vi "MethodSCRIPTExample.vi"() -> ()   [LabVIEW 2025]
uses:
  PalmSens/PalmSens.lvclass
  PalmSens/MeasurementResults.ctl
  PalmSens/LiveCurveResult.ctl
  C:/Users/stef/code/palmsenssdk/labview/PalmSens/Libraries/PalmSens.Core.Simplified.LabVIEW.dll
  PalmSens/Libraries/PalmSens.Core.Simplified.LabVIEW.dll
panel:
  out "Curves":T1
  out "MethodSCRIPT":refnum<k24>
  out "Array":string[](array[string])
  out "Is Measuring":bool
  in  "PalmSens.lvclass":refnum<class "PalmSens.lvclass">
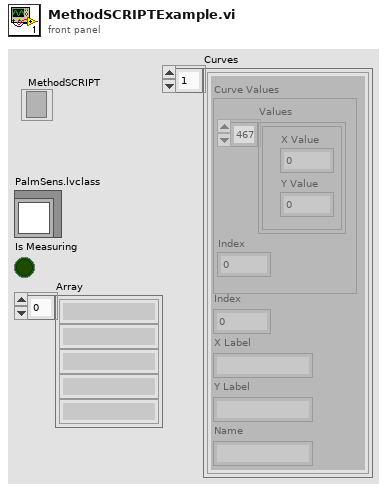
[diagram p1: front panel]
types:
  T1 = typedef "MeasurementResults.ctl" = T2[]
  T2 = typedef "LiveCurveResult.ctl" = cluster{"X Label":string, "Y Label":string, "Name":string, "Index":i16, "Curve Values":cluster{"Values":cluster{"X Value":dbl, "Y Value":dbl}[], "Index":i16}}
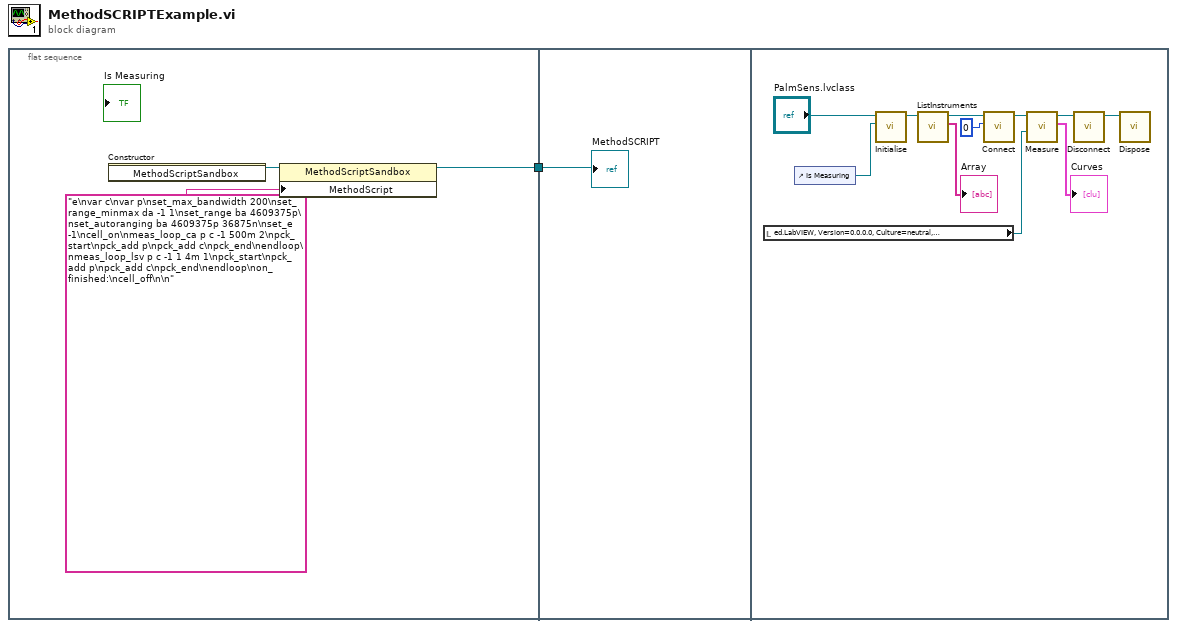
[diagram p0: block diagram]
diagram:
  n1 = flat-sequence {
    tunnel: [w2] -> w1
    tunnel: w1 -> [w5]
    frame #0 {
      n2 = constructor class="MethodScriptSandbox"() -> (reference out=w4:refnum<k24>)  [unwired: 3 in, 2 out]
      n3 = property class="MethodScriptSandbox"(reference=w4, "MethodScript"="e\nvar c\nvar p\nset_max_bandwidth 200\nset_range_minmax da -1 1\nset_range ba 4609375p\nset_autoranging ba 4609375p 36875n\nset_e -1\ncell_on\nmeas_loop_ca p c -1 500m 2\npck_start\npck_add p\npck_add c\npck_end\nendloop\nmeas_loop_lsv p c -1 1 4m 1\npck_start\npck_add p\npck_add c\npck_end\nendloop\non_finished:\ncell_off\n\n") -> (reference out=w2:refnum<k24>)  [unwired: 1 in, 1 out]
    }
    frame #1 {
      "MethodSCRIPT" <- w5
    }
    frame #2 {
      n4 = local read "MethodSCRIPT"() -> (w16:refnum<k24>)
      n5 = control-ref of="Is Measuring"() -> (w8:refnum<vi>)
      n6 = call-dynamic "Initialise.vi"("Is Measuring Refnum"=w8, "PalmSens in"="PalmSens.lvclass") -> ("PalmSens out"=w9:refnum<class "PalmSens.lvclass">)  [unwired: 8 in, 1 out]
      n7 = call-dynamic "ListInstruments.vi"("PalmSens in"=w9) -> ("Array"=→"Array":string[], "PalmSens out"=w11:refnum<class "PalmSens.lvclass">)  [unwired: 8 in, 1 out]
      n8 = call-dynamic "Connect.vi"("Instrument Index"=0, "PalmSens in"=w11) -> ("PalmSens out"=w13:refnum<class "PalmSens.lvclass">)  [unwired: 8 in, 1 out]
      n9 = call-dynamic "Measure.vi"("Method .NET Refnum"=w16, "PalmSens in"=w13) -> ("Curves"=→"Curves":T1, "PalmSens out"=w14:refnum<class "PalmSens.lvclass">)  [unwired: 2 in, 2 out]
      n10 = call-dynamic "Disconnect.vi"("PalmSens in"=w14) -> ("PalmSens out"=w12:refnum<class "PalmSens.lvclass">)  [unwired: 9 in, 1 out]
      n11 = call-dynamic "Dispose.vi"("PalmSens in"=w12) -> ()  [unwired: 9 in, 2 out]
    }
  }
